vi "InitializeLasers.vi"() -> (0 "error out":errorcluster, 3 "hALC_REV out":i32)   [LabVIEW 2015]
uses:
  <userlib>/AB_ALC_REV64/AB_ALC_REV64.lvlib
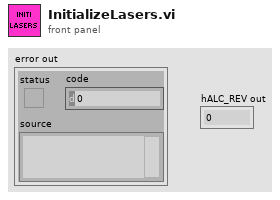
[diagram p1: front panel]
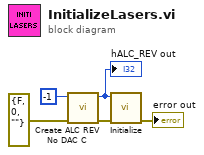
[diagram p0: block diagram]
diagram:
  n1 = call <userlib>:"Create ALC REV No DAC C.vi"("error in (no error)"=errorcluster {"status"=FALSE, "code"=0, "source"=""}, "hALC_REV"=-1) -> ("error out"=w4:errorcluster, "hALC_REV out"=w2:i32)  [unwired: 7 in, 1 out]
  "hALC_REV out" <- w2
  n2 = call <userlib>:"Initialize.vi"("error in (no error)"=w4, "hALC_REV_Laser"=w2) -> ("error out"=→"error out":errorcluster)  [unwired: 8 in, 1 out]
